vi "String description of single criteria.vi"(7 "Criteria":T1, 12 "User input":dbl) -> (8 "String":string, 10 "Immediate":bool)   [LabVIEW 2011]
uses:
  Single criteria cluster.ctl
  Criteria types.ctl
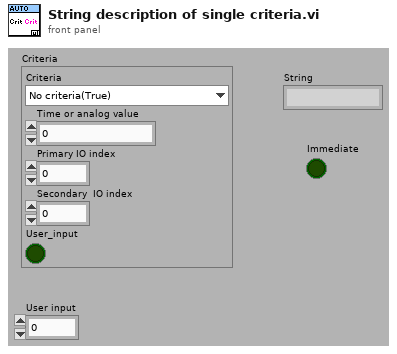
[diagram p1: front panel]
types:
  T1 = typedef "Single criteria cluster.ctl" = cluster{"Criteria":T2, "Time or analog value":dbl, "Primary IO index":i32, "Secondary  IO index":i32, "User_input":bool}
  T2 = typedef "Criteria types.ctl" = enum16{"No criteria(True)", "Time(s)", "Analog IO over", "Analog IO over or equal", "Analog IO under", "Analog IO under or equal", "Analog IO 1 minus Analog IO 2 over", "Digital IO True", "Digital IO False", "Operator approval"}
  T3 = typedef "Fixed Analog Channel Definition.ctl" = cluster{"ID":u16, "Name":string, "Quantity":T4, "Unit":string, "Maximum upd":T5, "Comment":string, "Help file Name":string, "Help file Section ":string, "Category":T6, "User adjustable Scaling":bool, "Default Scaling":T7, "Default Unit":i32, "Classification":T8}
  T4 = typedef "Quantity enum.ctl" = enum16{"NA", "Acceleration", "Angle", "Current", "Force", "Distance", "Pressure", "Resistance", "Rotational Speed", "Speed", "Temperature", "Tension", "Torque", "Voltage", "Weight"}
  T5 = typedef "Update frequensies.ctl" = enum16{"2 Hz", "1 Hz", "0.1 Hz"}
  T6 = typedef "Channel catagory Enum.ctl" = enum16{"No Category", "Power", "Temperature", "Pressure"}
  T7 = typedef "Scaling.ctl" = cluster{"Gain":dbl, "Offset":dbl}
  T8 = typedef "Channel Classification Enum.ctl" = enum16{"Basic", "Advanced", "Expert", "Unused"}
  T9 = typedef "Analog Var Disp 0 sif.ctl" = cluster{"Value":dbl, "Unit":string, "Status":T10}
  T10 = typedef "Status indicator Black Small.ctl" = u16
  T11 = typedef "Fixed Digital Channel Definition.ctl" = cluster{"ID":u16, "Name":string, "NA Text":string, "Off Text":string, "On Text":string, "Maximum upd":T5, "Comment":string, "Help file Name":string, "Help file Section ":string, "Catagory":T6, "In use":bool}
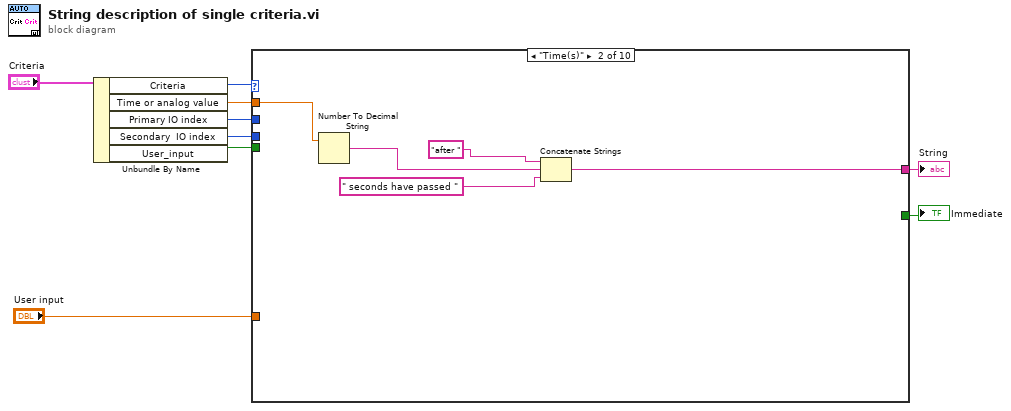
[diagram p0: block diagram]
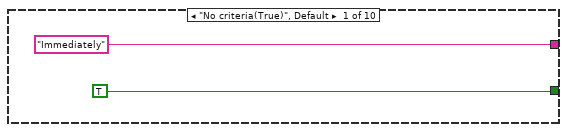
[diagram p2: hidden frame]
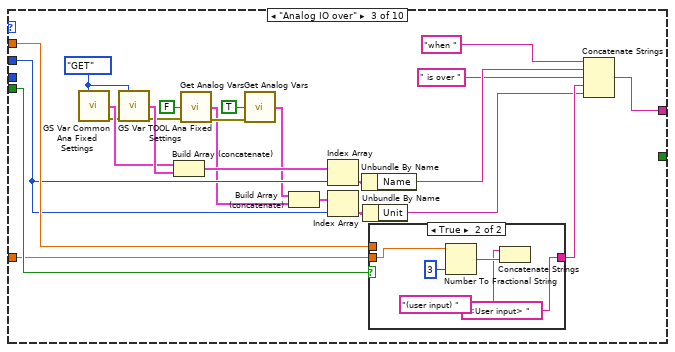
[diagram p3: hidden frame]
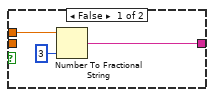
[diagram p4: hidden frame]
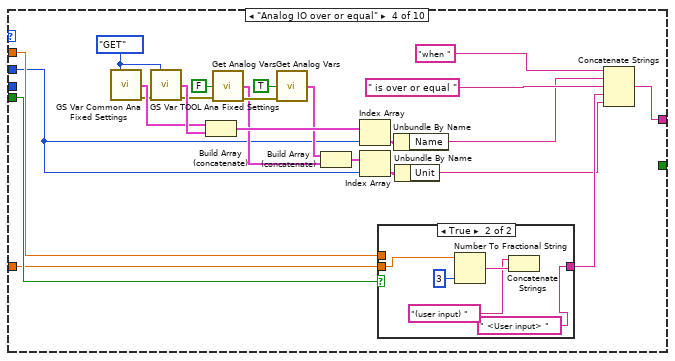
[diagram p5: hidden frame]
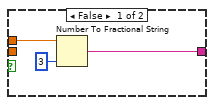
[diagram p6: hidden frame]
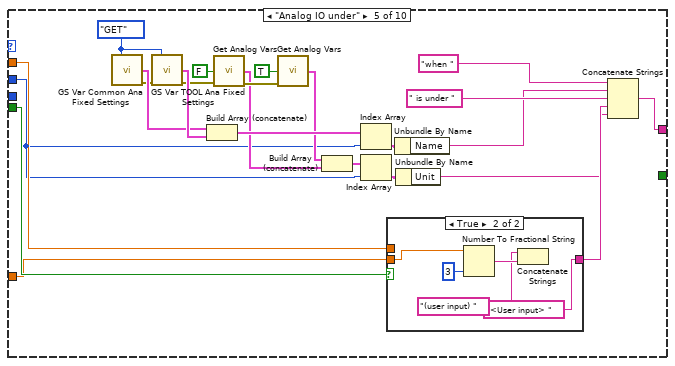
[diagram p7: hidden frame]
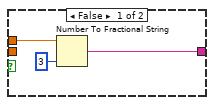
[diagram p8: hidden frame]
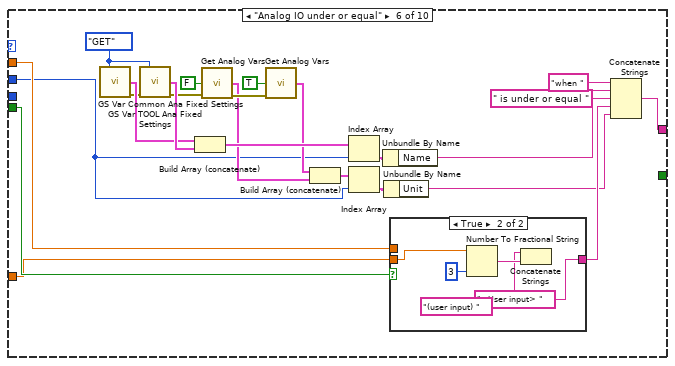
[diagram p9: hidden frame]
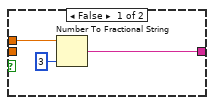
[diagram p10: hidden frame]
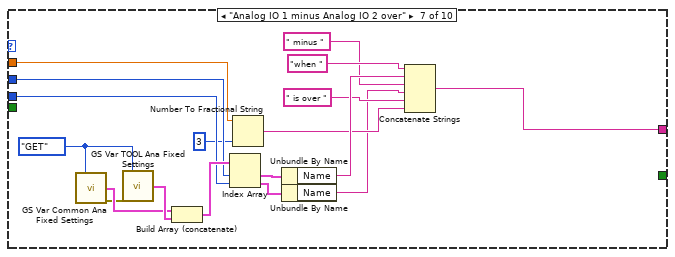
[diagram p11: hidden frame]
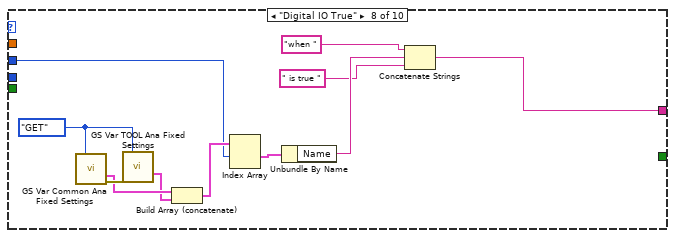
[diagram p12: hidden frame]
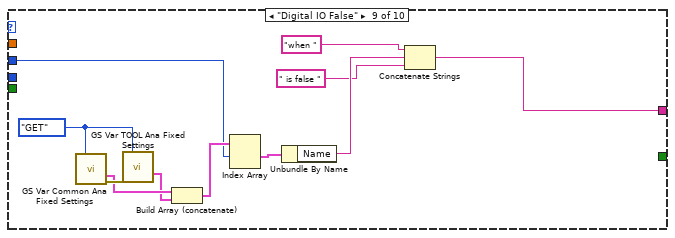
[diagram p13: hidden frame]
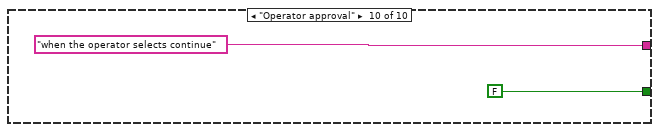
[diagram p14: hidden frame]
diagram:
  n1 = Unbundle By Name("Criteria") -> ("Criteria"=w5:T2, "Time or analog value"=w6:dbl, "Primary IO index"=w7:i32, "Secondary  IO index"=w8:i32, "User_input"=w1:bool)
  n2 = case shown="\"Time(s)\"" w5 {
    tunnel: w6 -> [_ w16 w31 w70 w100 w132 w152 _ _ _]
    tunnel: ["Immediately" w12 w29 w68 w102 w134 w150 w166 w177 "when the operator selects continue"] -> w9
    tunnel: w7 -> [_ _ w22 w49 w83 w113 w157 w170 w181 _]
    tunnel: w8 -> [_ _ _ _ _ _ w149 _ _ _]
    tunnel: [TRUE ("Immediate") _ _ _ _ _ _ _ _ FALSE ("Immediate")] -> w3
    tunnel: "User input" -> [_ _ w27 w66 w99 w131 _ _ _ _]
    tunnel: w1 -> [_ _ w28 w67 w101 w133 _ _ _ _]
    frame "No criteria(True)", Default {
    }
    frame "Time(s)" {
      n3 = Number To Decimal String(number=w16) -> (decimal integer string=w14:string)  [unwired: 1 in]
      n4 = Concatenate Strings("after " ("string"), w14, " seconds have passed " ("string")) -> (w12:string)
    }
    frame "Analog IO over" {
      w38 = enum16{"GET", "SET"}."GET" ("Action(GET)")
      n5 = call "GS Var Common Ana Fixed Settings.vi"("Action(GET)"=w38) -> ("Common Analog Var Fixed out"=w39:T3[], "error out"=w37:errorcluster)  [unwired: 12 in, 1 out]
      n6 = call "GS Var TOOL Ana Fixed Settings.vi"("Action(GET)"=w38, "error in (no error)"=w37) -> ("Tool Analog var Fixed out"=w40:T3[], "error out"=w23:errorcluster)  [unwired: 11 in, 1 out]
      n7 = Build Array (concatenate)(w39, w40) -> (w36:T3[])
      n8 = call "Get Analog Vars.vi"("Tool"=FALSE, "error in (no error)"=w23) -> ("Analog Vars"=w20:T9[], "error out"=w26:errorcluster)  [unwired: 7 in, 5 out]
      n9 = call "Get Analog Vars.vi"("Tool"=TRUE, "error in (no error)"=w26) -> ("Analog Vars"=w21:T9[])  [unwired: 7 in, 6 out]
      n10 = Build Array (concatenate)(w21, w20) -> (w19:T9[])
      n11 = Index Array(array=w36, index=w22) -> (element=w35:T3)
      n12 = Index Array(array=w19, index=w22) -> (element=w18:T9)
      n13 = Unbundle By Name(w35) -> ("Name"=w33:string)
      n14 = Unbundle By Name(w18) -> ("Unit"=w17:string)
      n15 = case shown="True" w28 {
        tunnel: w31 -> [w43 _]
        tunnel: [w42 "<User input> "] -> w30
        tunnel: w27 -> [_ w46]
        frame False {
          n16 = Number To Fractional String(number=w43, precision (6)=i16 3) -> (F-format string=w42:string)  [unwired: 2 in]
        }
        frame True {
          n17 = Number To Fractional String(number=w46, precision (6)=i16 3) -> (F-format string=w48:string)  [unwired: 2 in]
          n18 = Concatenate Strings("(user input) ", w48) -> ()  [unwired: 1 out]
        }
      }
      n19 = Concatenate Strings("when ", w33, " is over " ("string"), w30, w17) -> (w29:string)
    }
    frame "Analog IO over or equal" {
      w63 = enum16{"GET", "SET"}."GET" ("Action(GET)")
      n20 = call "GS Var Common Ana Fixed Settings.vi"("Action(GET)"=w63) -> ("Common Analog Var Fixed out"=w64:T3[], "error out"=w62:errorcluster)  [unwired: 12 in, 1 out]
      n21 = call "GS Var TOOL Ana Fixed Settings.vi"("Action(GET)"=w63, "error in (no error)"=w62) -> ("Tool Analog var Fixed out"=w65:T3[], "error out"=w56:errorcluster)  [unwired: 11 in, 1 out]
      n22 = Build Array (concatenate)(w64, w65) -> (w61:T3[])
      n23 = call "Get Analog Vars.vi"("Tool"=FALSE, "error in (no error)"=w56) -> ("Analog Vars"=w54:T9[], "error out"=w59:errorcluster)  [unwired: 7 in, 5 out]
      n24 = call "Get Analog Vars.vi"("Tool"=TRUE, "error in (no error)"=w59) -> ("Analog Vars"=w55:T9[])  [unwired: 7 in, 6 out]
      n25 = Build Array (concatenate)(w55, w54) -> (w53:T9[])
      n26 = Index Array(array=w61, index=w49) -> (element=w60:T3)
      n27 = Index Array(array=w53, index=w49) -> (element=w52:T9)
      n28 = case shown="True" w67 {
        tunnel: w70 -> [w75 _]
        tunnel: [w74 " <User input> "] -> w69
        tunnel: w66 -> [_ w78]
        frame False {
          n29 = Number To Fractional String(number=w75, precision (6)=i16 3) -> (F-format string=w74:string)  [unwired: 2 in]
        }
        frame True {
          n30 = Number To Fractional String(number=w78, precision (6)=i16 3) -> (F-format string=w80:string)  [unwired: 2 in]
          n31 = Concatenate Strings("(user input) ", w80) -> ()  [unwired: 1 out]
        }
      }
      n32 = Unbundle By Name(w60) -> ("Name"=w51:string)
      n33 = Unbundle By Name(w52) -> ("Unit"=w50:string)
      n34 = Concatenate Strings("when ", w51, " is over or equal " ("string"), w69, w50) -> (w68:string)
    }
    frame "Analog IO under" {
      w95 = enum16{"GET", "SET"}."GET" ("Action(GET)")
      n35 = call "GS Var Common Ana Fixed Settings.vi"("Action(GET)"=w95) -> ("Common Analog Var Fixed out"=w96:T3[], "error out"=w94:errorcluster)  [unwired: 12 in, 1 out]
      n36 = call "GS Var TOOL Ana Fixed Settings.vi"("Action(GET)"=w95, "error in (no error)"=w94) -> ("Tool Analog var Fixed out"=w97:T3[], "error out"=w88:errorcluster)  [unwired: 11 in, 1 out]
      n37 = Build Array (concatenate)(w96, w97) -> (w93:T3[])
      n38 = call "Get Analog Vars.vi"("Tool"=FALSE, "error in (no error)"=w88) -> ("Analog Vars"=w86:T9[], "error out"=w91:errorcluster)  [unwired: 7 in, 5 out]
      n39 = call "Get Analog Vars.vi"("Tool"=TRUE, "error in (no error)"=w91) -> ("Analog Vars"=w87:T9[])  [unwired: 7 in, 6 out]
      n40 = Build Array (concatenate)(w87, w86) -> (w85:T9[])
      n41 = Index Array(array=w93, index=w83) -> (element=w92:T3)
      n42 = Index Array(array=w85, index=w83) -> (element=w84:T9)
      n43 = case shown="True" w101 {
        tunnel: w100 -> [w107 _]
        tunnel: [w106 "<User input> "] -> w98
        tunnel: w99 -> [_ w110]
        frame False {
          n44 = Number To Fractional String(number=w107, precision (6)=i16 3) -> (F-format string=w106:string)  [unwired: 2 in]
        }
        frame True {
          n45 = Number To Fractional String(number=w110, precision (6)=i16 3) -> (F-format string=w112:string)  [unwired: 2 in]
          n46 = Concatenate Strings("(user input) ", w112) -> ()  [unwired: 1 out]
        }
      }
      n47 = Unbundle By Name(w92) -> ("Name"=w82:string)
      n48 = Unbundle By Name(w84) -> ("Unit"=w81:string)
      n49 = Concatenate Strings("when ", w82, " is under " ("string"), w98, w81) -> (w102:string)
    }
    frame "Analog IO under or equal" {
      w127 = enum16{"GET", "SET"}."GET" ("Action(GET)")
      n50 = call "GS Var Common Ana Fixed Settings.vi"("Action(GET)"=w127) -> ("Common Analog Var Fixed out"=w128:T3[], "error out"=w126:errorcluster)  [unwired: 12 in, 1 out]
      n51 = call "GS Var TOOL Ana Fixed Settings.vi"("Action(GET)"=w127, "error in (no error)"=w126) -> ("Tool Analog var Fixed out"=w129:T3[], "error out"=w120:errorcluster)  [unwired: 11 in, 1 out]
      n52 = Build Array (concatenate)(w128, w129) -> (w125:T3[])
      n53 = call "Get Analog Vars.vi"("Tool"=FALSE, "error in (no error)"=w120) -> ("Analog Vars"=w118:T9[], "error out"=w123:errorcluster)  [unwired: 7 in, 5 out]
      n54 = call "Get Analog Vars.vi"("Tool"=TRUE, "error in (no error)"=w123) -> ("Analog Vars"=w119:T9[])  [unwired: 7 in, 6 out]
      n55 = Build Array (concatenate)(w119, w118) -> (w117:T9[])
      n56 = Index Array(array=w125, index=w113) -> (element=w124:T3)
      n57 = Index Array(array=w117, index=w113) -> (element=w116:T9)
      n58 = Unbundle By Name(w124) -> ("Name"=w115:string)
      n59 = Unbundle By Name(w116) -> ("Unit"=w114:string)
      n60 = case shown="True" w133 {
        tunnel: w132 -> [w139 _]
        tunnel: [w138 "<User input> "] -> w130
        tunnel: w131 -> [_ w142]
        frame False {
          n61 = Number To Fractional String(number=w139, precision (6)=i16 3) -> (F-format string=w138:string)  [unwired: 2 in]
        }
        frame True {
          n62 = Number To Fractional String(number=w142, precision (6)=i16 3) -> (F-format string=w144:string)  [unwired: 2 in]
          n63 = Concatenate Strings("(user input) ", w144) -> ()  [unwired: 1 out]
        }
      }
      n64 = Concatenate Strings("when ", w115, " is under or equal " ("string"), w130, w114) -> (w134:string)
    }
    frame "Analog IO 1 minus Analog IO 2 over" {
      w160 = enum16{"GET", "SET"}."GET" ("Action(GET)")
      n65 = call "GS Var Common Ana Fixed Settings.vi"("Action(GET)"=w160) -> ("Common Analog Var Fixed out"=w161:T3[], "error out"=w159:errorcluster)  [unwired: 12 in, 1 out]
      n66 = call "GS Var TOOL Ana Fixed Settings.vi"("Action(GET)"=w160, "error in (no error)"=w159) -> ("Tool Analog var Fixed out"=w162:T3[])  [unwired: 11 in, 2 out]
      n67 = Build Array (concatenate)(w161, w162) -> (w158:T3[])
      n68 = Index Array(array=w158, index #1=w157, index #2=w149) -> (element #1=w156:T3, element #2=w148:T3)
      n69 = Number To Fractional String(number=w152, precision (6)=i16 3) -> (F-format string=w151:string)  [unwired: 2 in]
      n70 = Unbundle By Name(w156) -> ("Name"=w154:string)
      n71 = Unbundle By Name(w148) -> ("Name"=w146:string)
      n72 = Concatenate Strings("when ", w154, " minus " ("string"), w146, " is over " ("string"), w151) -> (w150:string)
    }
    frame "Digital IO True" {
      w173 = enum16{"GET", "SET"}."GET" ("Action(GET)")
      n73 = call "GS Var Common Ana Fixed Settings.vi"("Action(GET)"=w173) -> ("Common Digital var Fixed"=w165:T11[], "error out"=w172:errorcluster)  [unwired: 12 in, 1 out]
      n74 = call "GS Var TOOL Ana Fixed Settings.vi"("Action(GET)"=w173, "error in (no error)"=w172) -> ("Tool Digital Var Fixed out"=w164:T11[])  [unwired: 11 in, 2 out]
      n75 = Build Array (concatenate)(w165, w164) -> (w171:T11[])
      n76 = Index Array(array=w171, index #1=w170) -> (element #1=w169:T11)  [unwired: 1 in, 1 out]
      n77 = Unbundle By Name(w169) -> ("Name"=w167:string)
      n78 = Concatenate Strings("when ", w167, " is true " ("string")) -> (w166:string)
    }
    frame "Digital IO False" {
      w184 = enum16{"GET", "SET"}."GET" ("Action(GET)")
      n79 = call "GS Var Common Ana Fixed Settings.vi"("Action(GET)"=w184) -> ("Common Digital var Fixed"=w176:T11[], "error out"=w183:errorcluster)  [unwired: 12 in, 1 out]
      n80 = call "GS Var TOOL Ana Fixed Settings.vi"("Action(GET)"=w184, "error in (no error)"=w183) -> ("Tool Digital Var Fixed out"=w175:T11[])  [unwired: 11 in, 2 out]
      n81 = Build Array (concatenate)(w176, w175) -> (w182:T11[])
      n82 = Index Array(array=w182, index #1=w181) -> (element #1=w180:T11)  [unwired: 1 in, 1 out]
      n83 = Unbundle By Name(w180) -> ("Name"=w178:string)
      n84 = Concatenate Strings("when ", w178, " is false " ("string")) -> (w177:string)
    }
    frame "Operator approval" {
    }
  }
  "String" <- w9
  "Immediate" <- w3
